vi "TurnToAngleController.vi"(5 "MaxAccel":dbl, 7 "MaxVel":dbl, 8 "Reset":bool, 9 "Gains":T1={"FFV"=0.0032, "FFA"=0.0, "Vel PID"={"P"=0.0, "I"=0.0, "D"=0.0}} {"Vel PID"."D" format="%.3f"; "Vel PID"."I" format="%.3f"; "Vel PID"."P" format="%.3f"}, 10 "CurrentAngle":dbl, 11 "TargetAngle":dbl) -> (0 "Done":bool, 1 "Time Left":u32, 2 "RightPower":dbl, 3 "LeftPower":dbl, 4 "VelGraph":cluster{"Output":dbl, "dx/dt":dbl}(graph)={"Output"=47.4353047807108, "dx/dt"=76.52582126109495}, 6 "Pos":dbl(graph)=299.88802132939395)   [LabVIEW 2017]
panel:
  out "Power":dbl(graph)=299.88802132939395
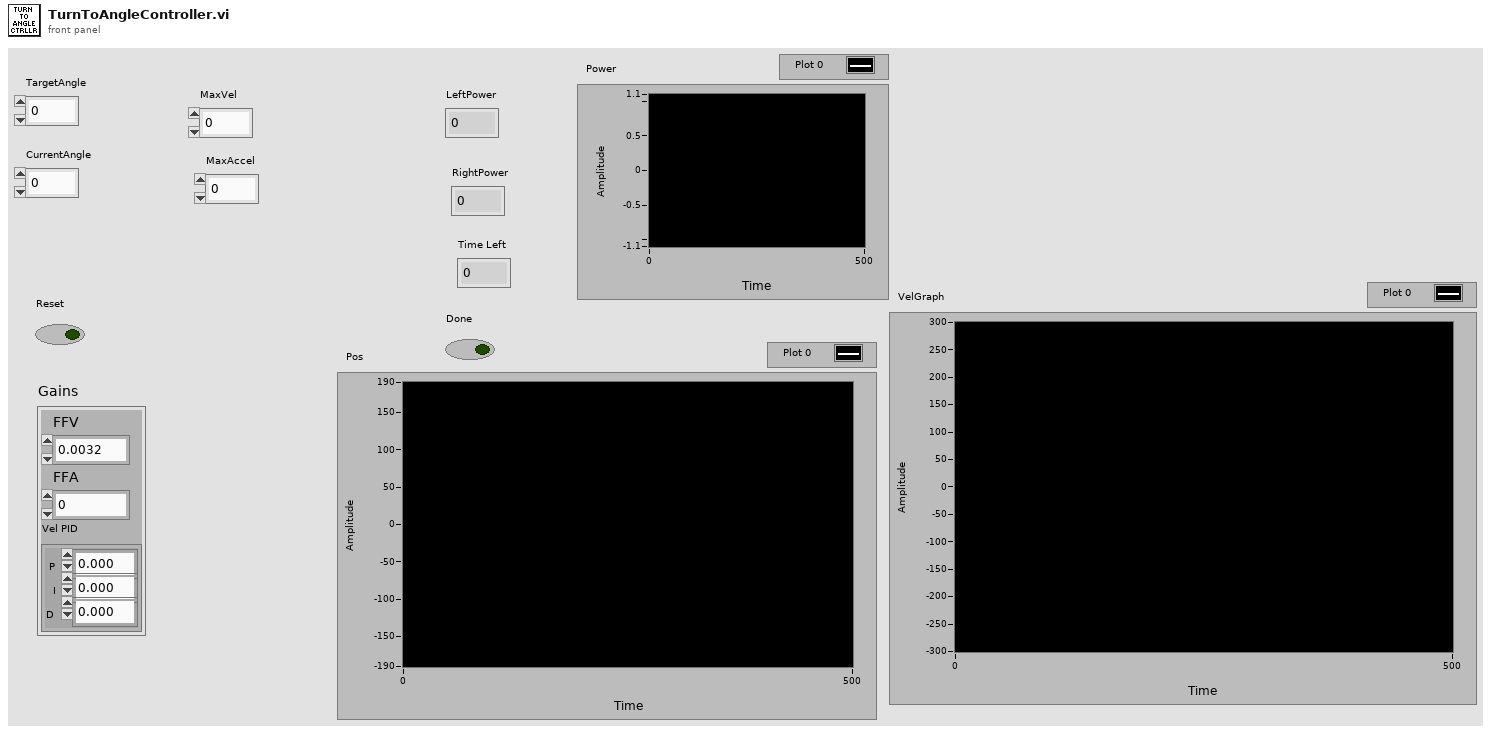
[diagram p1: front panel]
types:
  T1 = cluster{"FFV":dbl, "FFA":dbl, "Vel PID":cluster{"P":dbl, "I":dbl, "D":dbl}}
  T2 = cluster{"Profile":cluster{"Distances":dbl[], "Vels":dbl[]}, "CurrentAngle":dbl}
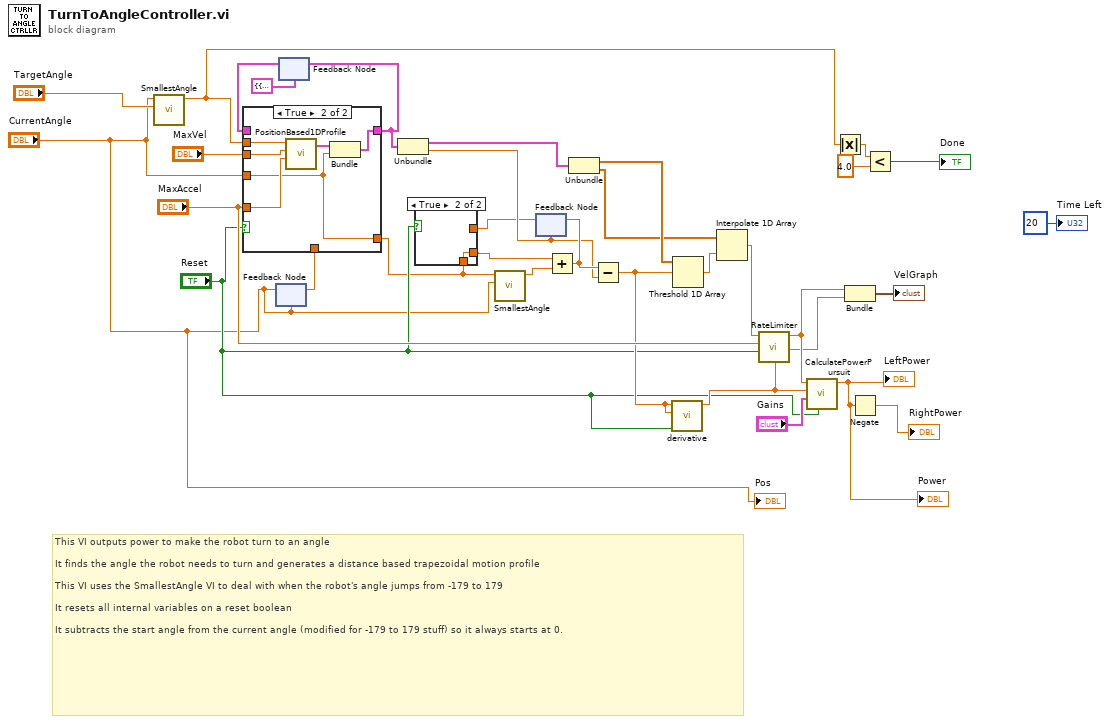
[diagram p0: block diagram]
diagram:
  # "This VI outputs power to make the robot turn to an angle\n\nIt finds the angle the robot needs to turn and generates a distance based trapezoidal motion profile\n\nThis VI uses the SmallestAngle VI to deal with when the robot's angle jumps from -179 to 179\n\nIt resets all internal variables on a reset boolean\n\nIt subtracts the start angle from the current angle (modified for -179 to 179 stuff) so it always starts at 0."
  n1 = call "SmallestAngle.vi"("Angle B"="TargetAngle", "Angle A"="CurrentAngle") -> ("Smallest A to B"=w11:dbl)  [unwired: 9 in]
  n2 = feedback #1("CurrentAngle") -> (w10:dbl)
  n3 = feedback-in #1("CurrentAngle") -> ()
  n4 = feedback #2(T2 {"Profile"={"Distances"=[], "Vels"=[]}, "CurrentAngle"=0.0}) -> (w30:T2)
  n5 = case shown="True" "Reset" {
    tunnel: w11 -> [_ w40]
    tunnel: "MaxVel" -> [_ w39]
    tunnel: "MaxAccel" -> [_ w38]
    tunnel: [w34 w37] -> w14
    tunnel: w30 -> [w34 _]
    tunnel: "CurrentAngle" -> [_ w35]
    tunnel: w10 -> [w33 _]
    tunnel: [w33 w35] -> w2
    frame False {
    }
    frame True {
      n6 = call "PositionBased1DProfile.vi"("MaxAccel"=w38, "MaxVel"=w39, "Distance"=w40) -> ("Profile"=w36:cluster{"Distances":dbl[], "Vels":dbl[]})  [unwired: 8 in]
      n7 = Bundle("Profile"=w36, "CurrentAngle"=w35) -> (w37:T2)  [unwired: 1 in]
    }
  }
  n8 = feedback-in #2(w14) -> ()
  n9 = Unbundle(w14) -> ("Profile"=w13:cluster{"Distances":dbl[], "Vels":dbl[]}, "CurrentAngle"=w8:dbl)
  n10 = call "SmallestAngle.vi"("Angle B"="CurrentAngle", "Angle A"=w2) -> ("Smallest A to B"=w12:dbl)  [unwired: 9 in]
  n11 = feedback #3(w8) -> (w4:dbl)
  n12 = case shown="True" "Reset" {
    tunnel: [w41 w42] -> w5
    tunnel: w4 -> [w41 _]
    tunnel: w2 -> [_ w42]
    frame False {
    }
    frame True {
    }
  }
  n13 = Add(x=w5, y=w12) -> (x+y=w9:dbl)
  n14 = feedback-in #3(w9) -> ()
  n15 = Unbundle(w13) -> ("Distances"=w29:dbl[], "Vels"=w28:dbl[])
  n16 = Subtract(x=w9, y=w8) -> (x-y=w6:dbl)
  n17 = call "derivative.vi"("Reset"="Reset", "Starting value"=w6, "x"=w6) -> ("dx/dt"=w7:dbl)  [unwired: 8 in]
  n18 = Threshold 1D Array(2:w6, 3:w29) -> (0:w27:dbl)  [unwired: 1 in]
  n19 = Interpolate 1D Array(1:w27, 2:w28) -> (0:w26:dbl)
  n20 = call "RateLimiter.vi"("Reset"="Reset", "Max dx/dt"="MaxAccel", "Input"=w26) -> ("Output"=w24:dbl)  [unwired: 8 in]
  n21 = call "CalculatePowerPursuit.vi"("Reset"="Reset", "Gains"="Gains", "Vel"=w7, "Target Vel"=w24) -> ("Power"=w17:dbl)  [unwired: 7 in]
  "LeftPower" <- w17
  "Power" <- w17
  n22 = Absolute Value(x=w11) -> (abs(x)=w22:dbl)
  n23 = Bundle("Output"=w24, "dx/dt"=w7) -> (→"VelGraph":cluster{"Output":dbl, "dx/dt":dbl})  [unwired: 1 in]
  n24 = Negate(x=w17) -> (-x=→"RightPower":dbl)
  n25 = Less?(x=w22, y=4.0) -> (x < y?=→"Done":bool)
  "Time Left" <- u32 20 ("Time Left")
  "Pos" <- "CurrentAngle"
